vi "Tutorial-Start.vi"() -> ()   [LabVIEW 2016]
panel:
  out "Connected to:":string
  in  "Available Devices":i32(listbox)
  in  "HSP eConArchive":bool
  in  "HSP FileTransfer":bool
  in  "HSP Buffer":bool
  in  "eGateUtility":bool
  in  "Configure":bool
  in  "Identify visually":bool
  in  "System Infos":bool
  in  "HSP Online":bool
  in  "Online ASCII":bool
  in  "Select Device":bool
  in  "Scan":bool
  # "Gantner-Instruments Tutorial - Ethernet"
  # "Online Data"
  # "Buffered Data"
  # "Configuration"
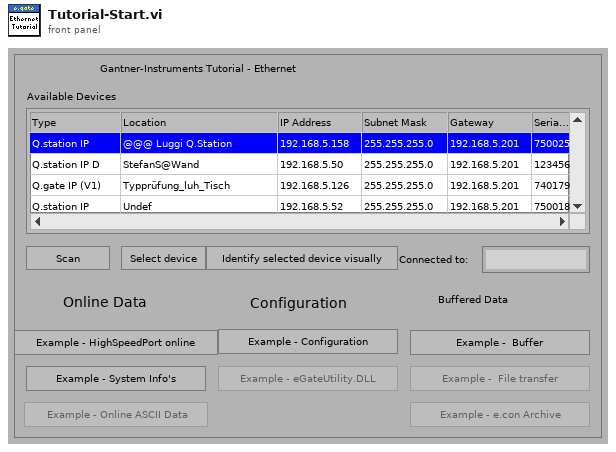
[diagram p1: front panel]
types:
  T1 = cluster{"Type":string, "Location":string, "Vendor":string, "MKCode":string, "DHCPMode":string, "IPAddress":string, "SubnetMask":string, "GatewayAddress":string, "MACAddress":string, "SerialNumber":string}
  T2 = cluster{"Type":string, "Location":string, "Vendor":string, "MKCode":string, "DHCPMode":string, "IPAddress":string, "SubnetMask":string, "GatewayAddress":string, "MACAddress":string, "SerialNumber":string}[]
  T3 = enum16{"idle", "scan", "select", "identify", "ascii_online", "hsp_online", "info_online", "config", "utility", "hsp_buffer", "hsp_file", "hsp_econArchive"}
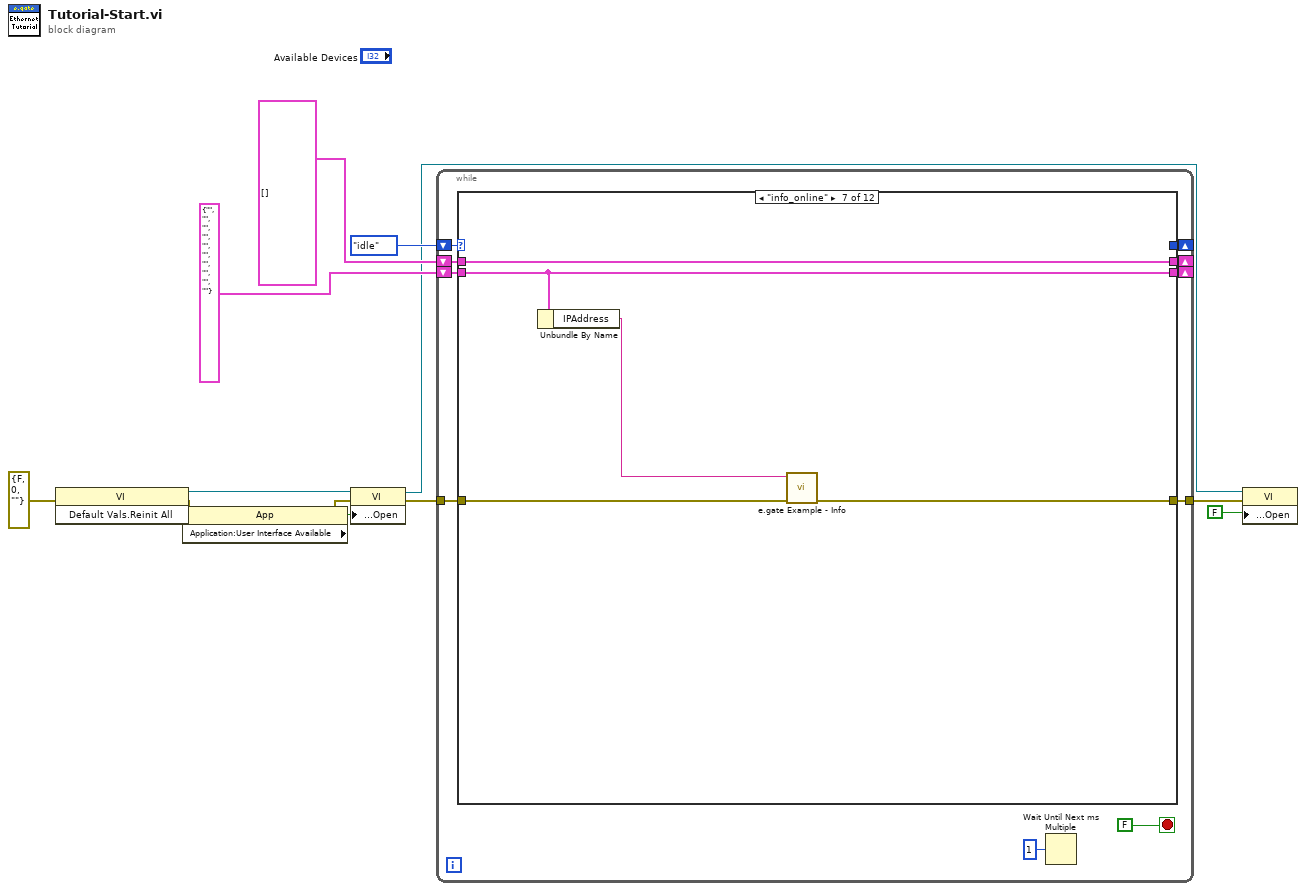
[diagram p0: block diagram]
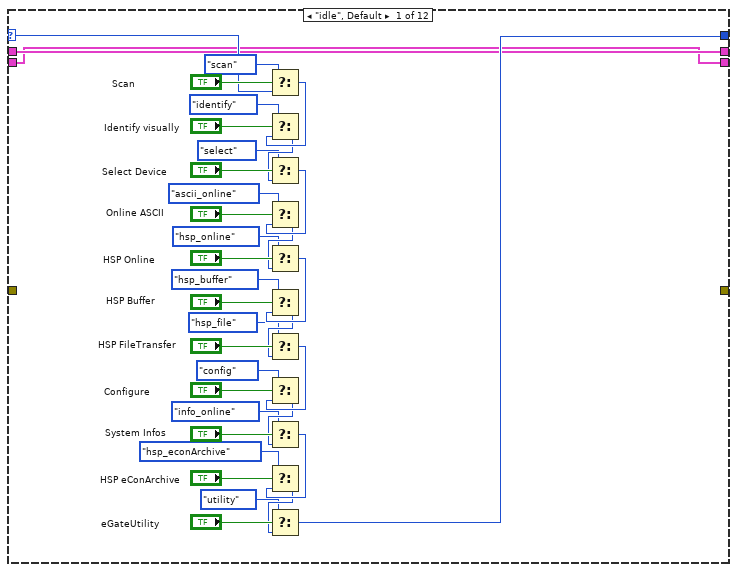
[diagram p2: hidden frame]
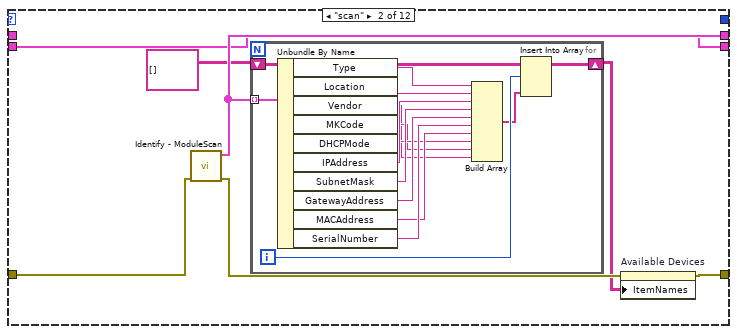
[diagram p3: hidden frame]
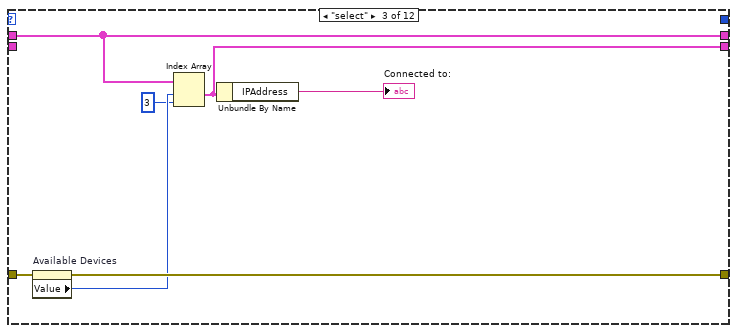
[diagram p4: hidden frame]
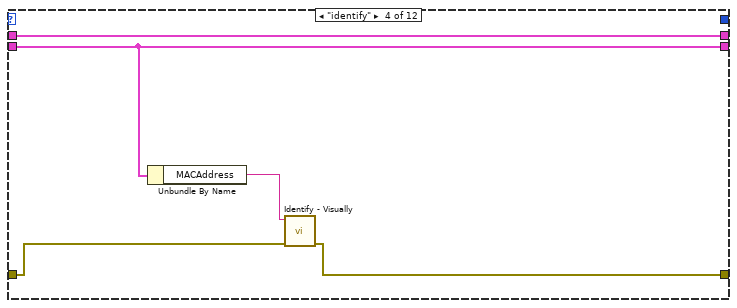
[diagram p5: hidden frame]
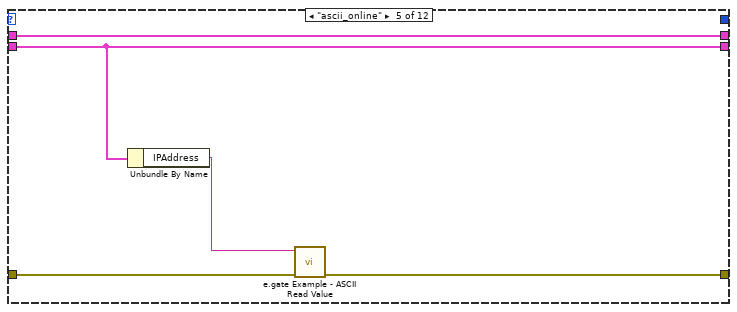
[diagram p6: hidden frame]
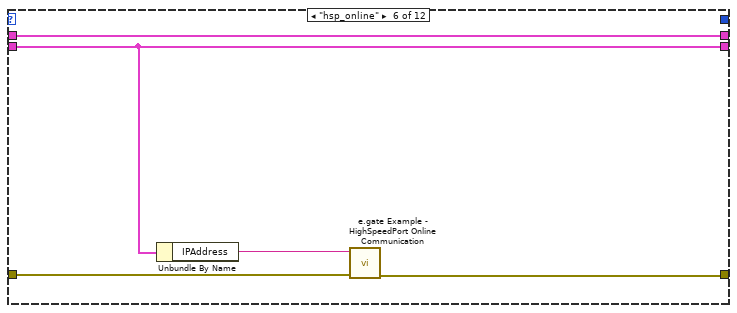
[diagram p7: hidden frame]
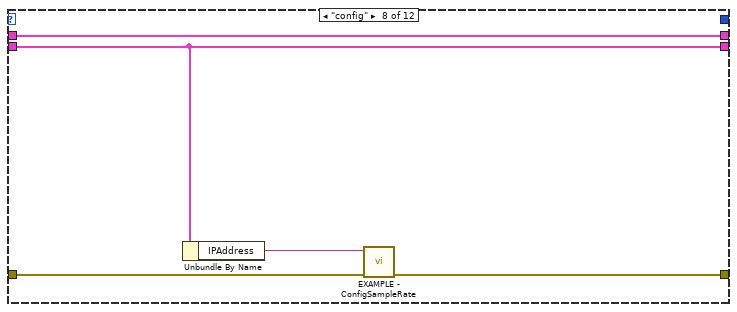
[diagram p8: hidden frame]
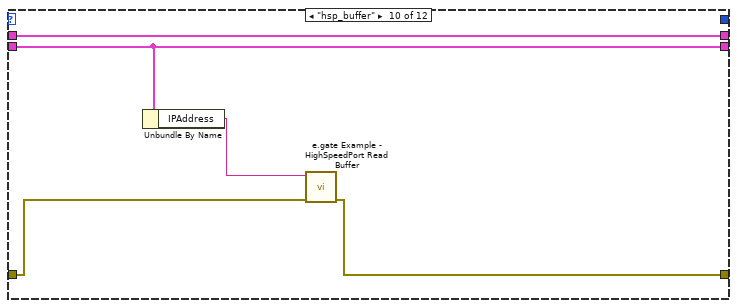
[diagram p10: hidden frame]
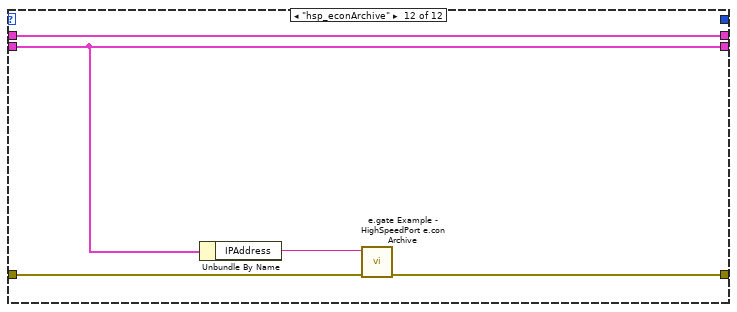
[diagram p12: hidden frame]
diagram:
  n1 = invoke class="VI" method="Default Vals.Reinit All"(error in=errorcluster {"status"=FALSE, "code"=0, "source"=""} ("Fehler (Eingang, kein Fehler)")) -> (reference out=w9:refnum<vi>, error out=w7:errorcluster)  [unwired: 2 in, 1 out]
  n2 = property class="App"(error in=w7) -> (error out=w6:errorcluster, "Application:User Interface Available"=w8:bool)  [unwired: 1 in, 1 out]
  n3 = property class="VI"(reference=w9, error in=w6, "Front Panel.Open"=w8) -> (reference out=w2:refnum<vi>, error out=w4:errorcluster)
  n4 = while {
    shift-right: [w21] -> _
    shift-left: T3."idle" ("State") -> [w22]
    tunnel: [w20] -> w3
    tunnel: w4 -> [w19]
    shift-right: [w18] -> _
    shift-left: T2 [] ("LifeList") -> [w17]
    shift-right: [w14] -> _
    shift-left: T1 {"Type"="", "Location"="", "Vendor"="", "MKCode"="", "DHCPMode"="", "IPAddress"="", "SubnetMask"="", "GatewayAddress"="", "MACAddress"="", "SerialNumber"=""} ("Info") -> [w13]
    stop <- FALSE stop-if-true
    n5 = case shown="\"info_online\"" w22 {
      selector: w22 -> [w47 _ _ _ _ _ _ _ _ _ _ _]
      tunnel: [w36 _ _ _ _ _ _ _ _ _ _ _] -> w21
      tunnel: [_ w63 w86 w90 w95 w100 w105 w108 _ w117 _ w124] -> w20
      tunnel: w19 -> [_ w65 w87 w91 w96 w101 w106 w109 _ w118 _ w125]
      tunnel: [w24 w64 w85 w92 w97 w102 w107 w112 w114 w119 w121 w126] -> w18
      tunnel: w17 -> [w24 _ w85 w92 w97 w102 w107 w112 w114 w119 w121 w126]
      tunnel: [w23 w59 w81 w89 w94 w99 w104 w111 w113 w115 w120 w123] -> w14
      tunnel: w13 -> [w23 w59 _ w89 w94 w99 w104 w111 w113 w115 w120 w123]
      frame "idle", Default {
        n6 = Select(t=T3."scan", s="Scan", f=w47) -> (s? t:f=w46:T3)
        n7 = Select(t=T3."identify", s="Identify visually", f=w46) -> (s? t:f=w41:T3)
        n8 = Select(t=T3."select", s="Select Device", f=w41) -> (s? t:f=w45:T3)
        n9 = Select(t=T3."ascii_online", s="Online ASCII", f=w45) -> (s? t:f=w40:T3)
        n10 = Select(t=T3."hsp_online", s="HSP Online", f=w40) -> (s? t:f=w44:T3)
        n11 = Select(t=T3."hsp_buffer", s="HSP Buffer", f=w44) -> (s? t:f=w39:T3)
        n12 = Select(t=T3."hsp_file", s="HSP FileTransfer", f=w39) -> (s? t:f=w43:T3)
        n13 = Select(t=T3."config", s="Configure", f=w43) -> (s? t:f=w38:T3)
        n14 = Select(t=T3."info_online", s="System Infos", f=w38) -> (s? t:f=w42:T3)
        n15 = Select(t=T3."hsp_econArchive", s="HSP eConArchive", f=w42) -> (s? t:f=w37:T3)
        n16 = Select(t=T3."utility", s="eGateUtility", f=w37) -> (s? t:f=w36:T3)
      }
      frame "scan" {
        n17 = call "Identify - ModuleScan.vi"("Fehler (Eingang, kein Fehler)"=w65) -> ("Fehler (Ausgang)"=w62:errorcluster, "LifeList"=w64:T2)  [unwired: 9 out]
        n18 = for {
          tunnel: w64 -> [w80] mode=indexing
          shift-right: [w77] -> w60
          shift-left: string[][] [] ("Objektnamen") -> [w79]
          i -> [w78]
          n19 = Unbundle By Name(w80) -> ("Type"=w75:string, "Location"=w74:string, "Vendor"=w66:string, "MKCode"=w67:string, "DHCPMode"=w68:string, "IPAddress"=w73:string, "SubnetMask"=w72:string, "GatewayAddress"=w71:string, "MACAddress"=w69:string, "SerialNumber"=w70:string)
          n20 = Build Array(w75, w74, w73, w72, w71, w70, w69, w68, w67, w66) -> (w76:string[])
          n21 = Insert Into Array(array=w79, index (row)=w78, new element=w76) -> (w77:string[][])  [unwired: 1 in]
        }
        n22 = property on="Available Devices" class="MCListbox (严格)"(error in=w62, "ItemNames"=w60) -> (error out=w63:errorcluster)  [unwired: 1 in, 1 out]
      }
      frame "select" {
        n23 = property on="Available Devices" class="MCListbox (严格)"(error in=w87) -> (error out=w86:errorcluster, "Value"=w84:i32)  [unwired: 1 in, 1 out]
        n24 = Index Array(array=w85, index #1=w84, index #2=3 ("Index")) -> (element #1=w81:T1)  [unwired: 1 out]
        n25 = Unbundle By Name(w81) -> ("IPAddress"=→"Connected to:":string)
      }
      frame "identify" {
        n26 = Unbundle By Name(w89) -> ("MACAddress"=w88:string)
        n27 = call "Identify - Visually.vi"("Fehler (Eingang, kein Fehler)"=w91, "MACAddress"=w88) -> ("Fehler (Ausgang)"=w90:errorcluster)  [unwired: 9 out]
      }
      frame "ascii_online" {
        n28 = Unbundle By Name(w94) -> ("IPAddress"=w93:string)
        n29 = call "e.gate Example - ASCII Read Value.vi"("Fehler (Eingang, kein Fehler)"=w96, "IP Address"=w93) -> ("error out"=w95:errorcluster)  [unwired: 9 out]
      }
      frame "hsp_online" {
        n30 = Unbundle By Name(w99) -> ("IPAddress"=w98:string)
        n31 = call "e.gate Example - HighSpeedPort Online Communication.vi"("Fehler (Eingang, kein Fehler)"=w101, "IP Address"=w98) -> ("error out"=w100:errorcluster)  [unwired: 9 out]
      }
      frame "info_online" {
        n32 = Unbundle By Name(w104) -> ("IPAddress"=w103:string)
        n33 = call "e.gate Example - Info.vi"("error in (no error)"=w106, "IP Address"=w103) -> ("error out"=w105:errorcluster)  [unwired: 9 out]
      }
      frame "config" {
        n34 = Unbundle By Name(w111) -> ("IPAddress"=w110:string)
        n35 = call "EXAMPLE - ConfigSampleRate.vi"("Fehler (Eingang, kein Fehler)"=w109, "IP"=w110) -> ("error out"=w108:errorcluster)  [unwired: 9 out]
      }
      frame "utility" {
      }
      frame "hsp_buffer" {
        n36 = Unbundle By Name(w115) -> ("IPAddress"=w116:string)
        n37 = call "e.gate Example - HighSpeedPort Read Buffer.vi"("Fehler (Eingang, kein Fehler)"=w118, "IP Address"=w116) -> ("error out"=w117:errorcluster)  [unwired: 9 out]
      }
      frame "hsp_file" {
      }
      frame "hsp_econArchive" {
        n38 = Unbundle By Name(w123) -> ("IPAddress"=w122:string)
        n39 = call "e.gate Example - HighSpeedPort e.con Archive.vi"("Fehler (Eingang, kein Fehler)"=w125, "IP Address"=w122) -> ("Fehler (Ausgang)"=w124:errorcluster)  [unwired: 9 out]
      }
    }
    n40 = Wait Until Next ms Multiple(millisecond multiple=u32 1 ("Vielfache von ms")) -> ()  [unwired: 1 out]
  }
  n41 = property class="VI"(reference=w2, error in=w3, "Front Panel.Open"=FALSE ("Frontpanel-Fenster:Öffnen")) -> ()  [unwired: 2 out]
